vi "GetType&ID.vi"(8 "Error In":errorcluster, 10 "Plugin reference out":refnum<class "ModuleAdmin.lvclass">, 11 "NHRGridSim in":refnum<class "NHRGridSim.lvclass">) -> (0 "Error Out":errorcluster, 1 "Cluster":T1, 2 "reference out":refnum<class "ModuleAdmin.lvclass">, 3 "NHRGridSim out":refnum<class "NHRGridSim.lvclass">)   [LabVIEW 2018, in "AcPwrPlugins.lvlib" / "NHRGridSim.lvclass"]
uses:
  NHRGridSim.lvclass
  <userlib>/NIST/ModuleAdminLib/ModuleAdmin/ModuleAdmin.lvclass
  AcPwrBaseClass/AcPwrBase.lvclass
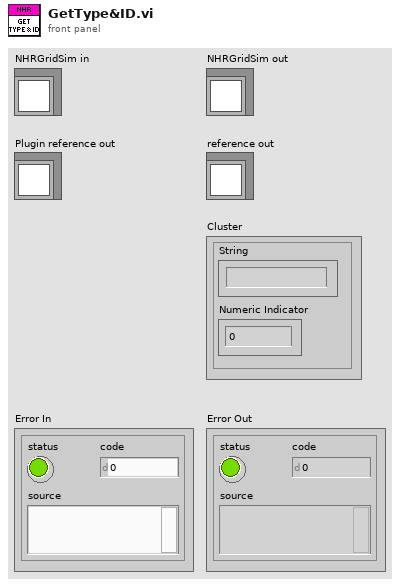
[diagram p1: front panel]
types:
  T1 = cluster{"String":string, "Numeric Indicator":i32}
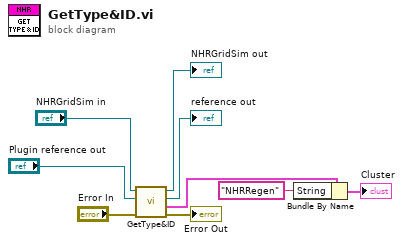
[diagram p0: block diagram]
diagram:
  n1 = call-parent "GetType&ID.vi"("Error In"="Error In", "Plugin reference out"="Plugin reference out", "AcPwrBase in"="NHRGridSim in") -> ("Error Out"=→"Error Out":errorcluster, "Cluster"=w1:T1, "reference out"=→"reference out":refnum<class "ModuleAdmin.lvclass">, "AcPwrBase out"=→"NHRGridSim out":refnum<class "NHRGridSim.lvclass">)  [unwired: 5 in]
  n2 = Bundle By Name(cluster=w1, "String"="NHRRegen") -> (→"Cluster":T1)
